vi "Open File.vi"(8 "error in (no error)":errorcluster, 11 "Path":path) -> (0 "error out":errorcluster={"status"=TRUE, "code"=4, "source"="Set File Position in Read IFDO.vi->Read Page Info.vi->TIFF Reader.lvclass:Open File.vi<APPEND>\nC:\\Users\\kleins\\Desktop\\4.0.stl"}, 2 "N Pages":i32=1, 3 "TIFF Reader.lvclass":refnum<class "TIFF Reader.lvclass">)   [LabVIEW 2020, in "LV Tiff.lvlib" / "TIFF Reader.lvclass"]
uses:
  TIFF Reader.lvclass
  TIFF Reader.lvclass/TIFF Reader.ctl
  LV Tiff.lvlib
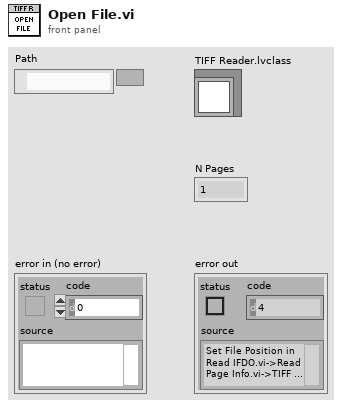
[diagram p1: front panel]
types:
  T1 = enum16{"big-endian, network order", "native, host order", "little-endian"}
  T2 = typedef "LV Tiff.lvlib/Tiff Data Type.ctl" = enum16{"Null", "BYTE", "ASCII", "SHORT", "LONG", "RATIONAL", "SBYTE", "UNDEFINE", "SSHORT", "SLONG", "SRATIONAL", "FLOAT", "DOUBLE"}
  T3 = cluster{i32, "Array":cluster{"TagID":u16, "DataType":T2, "DataCount":u32, "DataOffset":u32}[], "IFDOffset":u32}[]
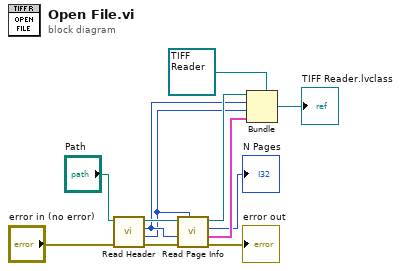
[diagram p0: block diagram]
diagram:
  n1 = call "Read Header.vi"("error in"="error in (no error)", "Path"="Path") -> ("error out"=w9:errorcluster, "IFDOffset"=w4:u32, "Tiff Bitness"=w5:T1, "refnum out"=w8:refnum<file>)  [unwired: 6 in]
  n2 = call "Read Page Info.vi"("IFDOffset"=w4, "error in (no error)"=w9, "Tiff Bitness"=w5, "Byte Stream File in"=w8) -> ("error in (no error) 2"=→"error out":errorcluster, "Page Info"=w3:T3, "N Pages"=→"N Pages":i32, "Byte Stream File out"=w6:refnum<file>)  [unwired: 4 in]
  n3 = Bundle(cluster=refnum<class "TIFF Reader.lvclass"> refnum ("TIFF Reader in"), w6, w5, w4, w3) -> (→"TIFF Reader.lvclass":refnum<class "TIFF Reader.lvclass">)
